vi "Read Identity.vi"(8 "error in (no error)":errorcluster, 11 "VISA resource name in":refnum<visa-resource-name>) -> (0 "error out":errorcluster, 2 "Identity":T1, 3 "VISA resource name":refnum<visa-resource-name>)   [LabVIEW 2023, in "CTI-Visa.lvlib"]
uses:
  CTI-Visa.lvlib
  Identity.ctl
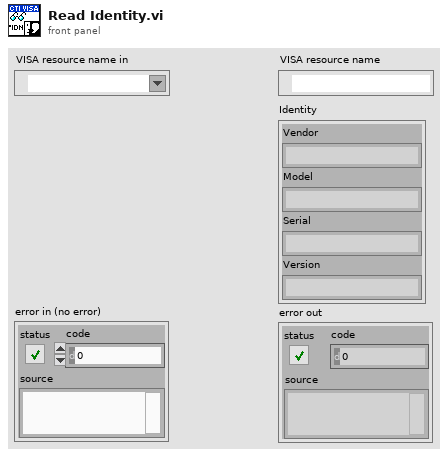
[diagram p1: front panel]
types:
  T1 = typedef "CTI-Visa.lvlib/Identity.ctl" = cluster{"Vendor":string, "Model":string, "Serial":string, "Version":string}
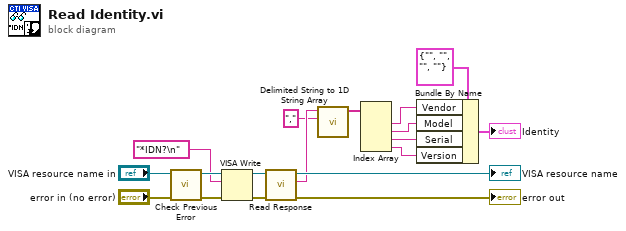
[diagram p0: block diagram]
diagram:
  n1 = call "Check Previous Error.vi"("error in (no error)"="error in (no error)", "VISA resource name in"="VISA resource name in") -> ("error out"=w17:errorcluster, "VISA resource name"=w14:refnum<visa-resource-name>)  [unwired: 8 in]
  n2 = VISA Write(VISA resource name=w14, write buffer="*IDN?\n", error in (no error)=w17) -> (VISA resource name out=w12:refnum<visa-resource-name>, error out=w18:errorcluster)  [unwired: 1 out]
  n3 = call "Read Response.vi"("error in (no error)"=w18, "VISA resource name in"=w12) -> ("error out"=→"error out":errorcluster, "Response"=w9:string, "VISA resource name"=→"VISA resource name":refnum<visa-resource-name>)  [unwired: 7 in]
  n4 = call <vilib>:"Delimited String to 1D String Array.vi"("delimiter"=",", "delimited string"=w9) -> ("string array"=w7:string[])  [unwired: 9 in]
  n5 = Index Array(array=w7) -> (element #1=w4:string, element #2=w3:string, element #3=w2:string, element #4=w1:string)  [unwired: 4 in]
  n6 = Bundle By Name(cluster=T1 {"Vendor"="", "Model"="", "Serial"="", "Version"=""} ("Identity"), "Vendor"=w4, "Model"=w3, "Serial"=w2, "Version"=w1) -> (→"Identity":T1)
